vi "drivetrain_drive_speed_store.vi"(9 "Write Thread":T1, 10 "data_store_mode":enum16{"Set", "Get"}(ring), 11 "drive data":cluster{"Left":dbl, "Right":dbl}) -> (2 "lock thread":T1, 3 "drive data out":cluster{"Left":dbl, "Right":dbl})   [LabVIEW 2011]
uses:
  drivetrain_drive_write_thread.ctl
panel:
  in  "Timeout":u32=51
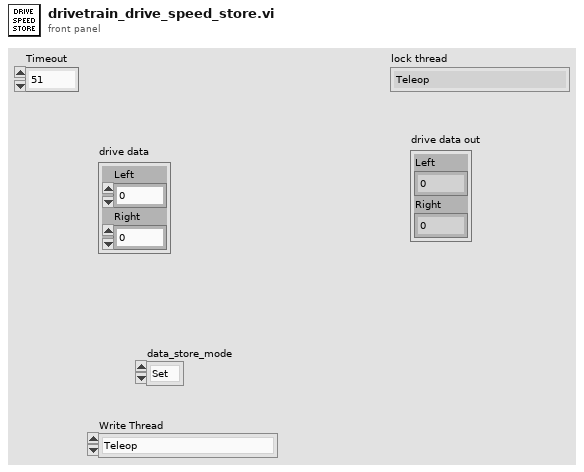
[diagram p1: front panel]
types:
  T1 = typedef "drivetrain_drive_write_thread.ctl" = enum16{"Teleop", "Script Engine - Autonomous", "Script Engine - Sequence"}
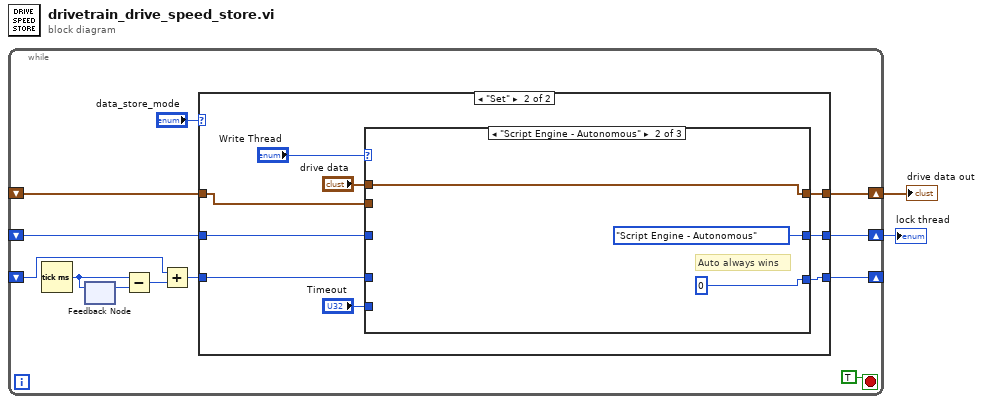
[diagram p0: block diagram]
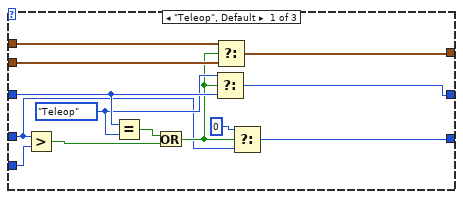
[diagram p3: hidden frame]
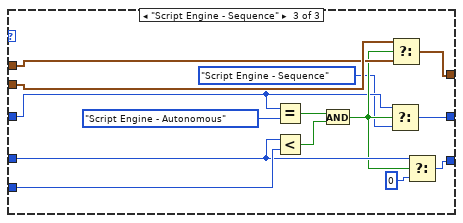
[diagram p4: hidden frame]
diagram:
  n1 = while {
    shift-right: [w12] -> w2
    shift-left: _ -> [w11]
    shift-right: [w4] -> w1
    shift-left: _ -> [w3]
    shift-right: [w6] -> _
    shift-left: _ -> [w8]
    stop <- TRUE stop-if-true
    n2 = Tick Count (ms)() -> (millisecond timer value=w10:u32)
    n3 = feedback-in #1(w10) -> ()
    n4 = feedback #1() -> (w9:u32)  [unwired: 1 in]
    n5 = Subtract(x=w10, y=w9) -> (x-y=w7:u32)
    n6 = Add(x=w8, y=w7) -> (x+y=w5:u32)
    n7 = case shown="\"Set\"" "data_store_mode" {
      tunnel: [w17 w24] -> w12
      tunnel: w11 -> [w17 w25]
      tunnel: [w16 w22] -> w6
      tunnel: w5 -> [w16 w19]
      tunnel: [w15 w21] -> w4
      tunnel: w3 -> [w15 w20]
      frame "Get", Default {
      }
      frame "Set" {
        n8 = case shown="\"Script Engine - Autonomous\"" "Write Thread" {
          tunnel: w25 -> [w35 _ w52]
          tunnel: [w34 w42 w50] -> w24
          tunnel: "drive data" -> [w36 w42 w51]
          tunnel: [w27 u32 0 w48] -> w22
          tunnel: [w33 drivetrain_drive_write_thread."Script Engine - Autonomous" ("Write Thread") w44] -> w21
          tunnel: w20 -> [w32 _ w45]
          tunnel: w19 -> [w29 _ w49]
          tunnel: "Timeout" -> [w39 _ w55]
          frame "Teleop", Default {
            w31 = drivetrain_drive_write_thread."Teleop" ("y")
            n9 = Greater?(x=w29, y=w39) -> (0:w37:bool)
            n10 = Equal?(x=w32, y=w31) -> (x = y?=w38:bool)
            n11 = Or(x=w38, y=w37) -> (x .or. y?=w30:bool)
            n12 = Select(t=w31, s=w30, f=w32) -> (s? t:f=w33:T1)
            n13 = Select(t=w36, s=w30, f=w35) -> (s? t:f=w34:cluster{"Left":dbl, "Right":dbl})
            n14 = Select(t=u32 0, s=w30, f=w29) -> (s? t:f=w27:u32)
          }
          frame "Script Engine - Autonomous" {
            # "Auto always wins"
          }
          frame "Script Engine - Sequence" {
            n15 = Equal?(x=w45, y=drivetrain_drive_write_thread."Script Engine - Autonomous") -> (x = y?=w54:bool)
            n16 = Less?(x=w49, y=w55) -> (x < y?=w53:bool)
            n17 = And(x=w54, y=w53) -> (x .and. y?=w46:bool)
            n18 = Select(t=w45, s=w46, f=drivetrain_drive_write_thread."Script Engine - Sequence") -> (s? t:f=w44:T1)
            n19 = Select(t=w52, s=w46, f=w51) -> (s? t:f=w50:cluster{"Left":dbl, "Right":dbl})
            n20 = Select(t=w49, s=w46, f=u32 0) -> (s? t:f=w48:u32)
          }
        }
      }
    }
  }
  "drive data out" <- w2
  "lock thread" <- w1
